vi "CaculateWaitingTimeForAlbum.vi"(9 "CurrentIndex":dbl=60000.0 format="%#_13g", 10 "ExpIncreaseEn?":bool=TRUE, 11 "Config":T1 {"Hardware Configuration"."Lasers Configuration"."SettingValues"."785 Power" format="%.1f"; "Hardware Configuration"."Lasers Configuration"."SettingValues"."647 Power" format="%.1f"; "Hardware Configuration"."Lasers Configuration"."SettingValues"."561 Power" format="%.1f"}) -> (1 "AcqTime/ms":dbl, 2 "AcqTime/min":dbl, 3 "Config 2":T1 {"Hardware Configuration"."Lasers Configuration"."SettingValues"."785 Power" format="%.1f"; "Hardware Configuration"."Lasers Configuration"."SettingValues"."647 Power" format="%.1f"; "Hardware Configuration"."Lasers Configuration"."SettingValues"."561 Power" format="%.1f"})   [LabVIEW 2019]
uses:
  Settings/System Running Settings.ctl
  Support/Hardware Configuration.ctl
  Support/Camera Configuration.ctl
  C:/RM21-MMicrosopeSource/HardwareAdapter/Camera/Dependencies/PVCamNET.dll
  Dependencies/PVCamNET.dll
  <vilib>/vision/Image Controls.llb/IMAQ Image.ctl
  C:/RM21-MMicrosopeSource/HardwareAdapter/Lasers/Dependencies/Oxxius_Boxx.dll
  Lasers/Dependencies/Oxxius_Boxx.dll
  Logging/Logging Configuration.ctl
  Controls/DeviceStatusCtl.ctl
  Controls/CallBack Refs.ctl
  Logging/Logging.lvlib
  Settings/Settings.lvlib
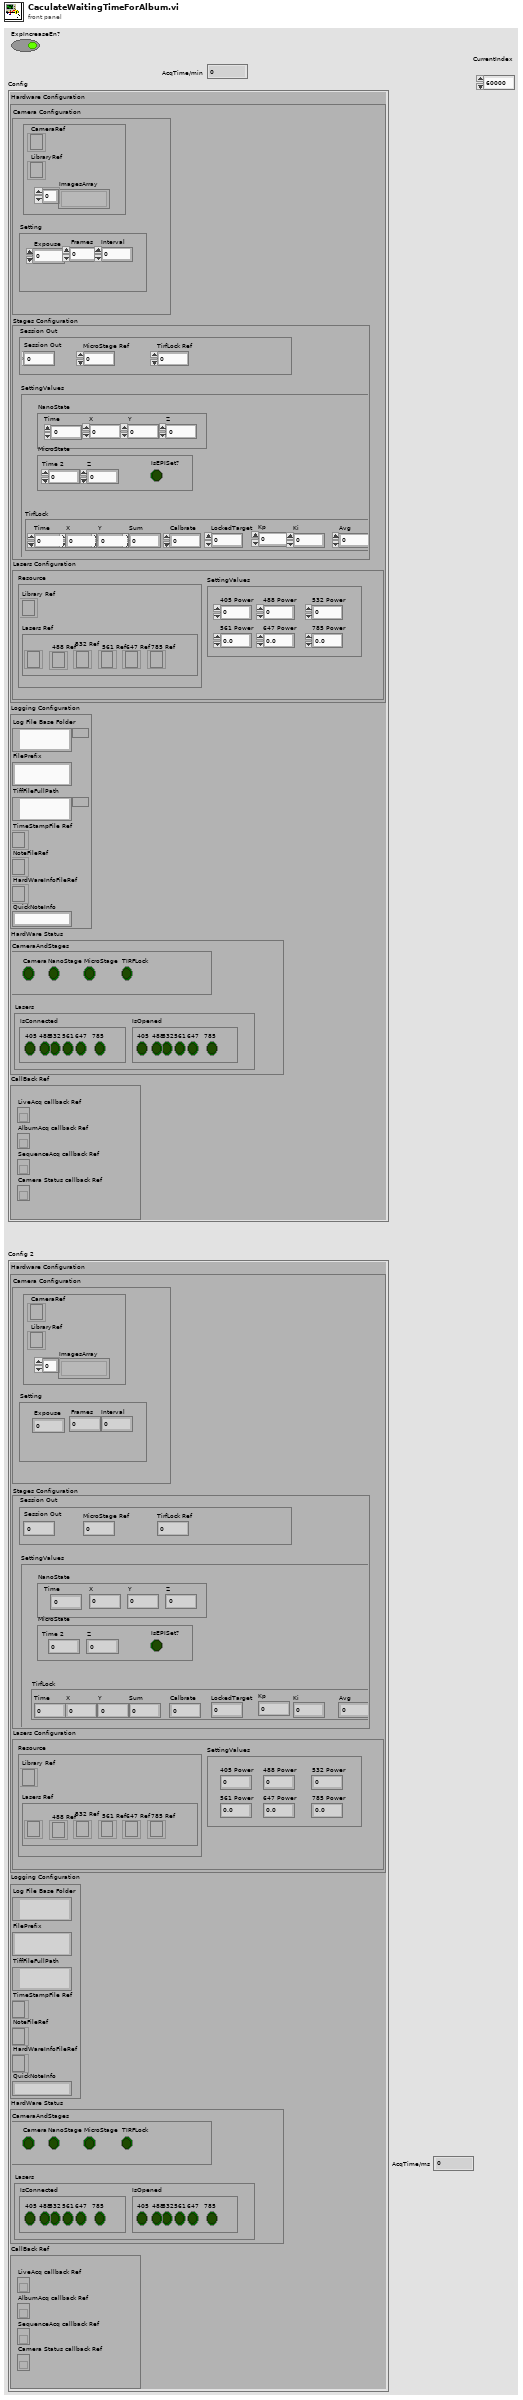
[diagram p1: front panel]
types:
  T1 = typedef "Settings.lvlib/System Running Settings.ctl" = cluster{"Hardware Configuration":T2, "Logging Configuration":T5, "HardWare Status":cluster{"CameraAndStages":T6, "Lasers":cluster{"IsConnected":cluster{"405":bool, "488":bool, "532":bool, "561":bool, "647":bool, "785":bool}, "IsOpened":cluster{"405":bool, "488":bool, "532":bool, "561":bool, "647":bool, "785":bool}}}, "CallBack Ref":T7}
  T2 = typedef "Hardware Configuration.ctl" = cluster{"Camera Configuration":T3, "Stages Configuration":cluster{"Resource":cluster{"NanoStage Ref":i32, "MicroStage Ref":i32, "TirfLock Ref":i32}, "SettingValues":cluster{"NanoState":cluster{"Time":dbl, "X":dbl, "Y":dbl, "Z":dbl}, "MicroState":cluster{"Time 2":dbl, "Z":dbl, "IsEPISet?":bool}, "TirfLock":cluster{"Time":dbl, "X":dbl, "Y":dbl, "Sum":dbl, "Calbrate":dbl, "LockedTarget":dbl, "Kp":dbl, "Ki":dbl, "Avg":dbl}}}, "Lasers Configuration":cluster{"SettingValues":cluster{"405 Power":sgl, "488 Power":sgl, "532 Power":sgl, "561 Power":sgl, "647 Power":sgl, "785 Power":sgl}, "Resource":cluster{"Library Ref":refnum<k24>, "Lasers Ref":cluster{"405 Ref":refnum<k24>, "488 Ref":refnum<k24>, "532 Ref":refnum<k24>, "561 Ref":refnum<k24>, "647 Ref":refnum<k24>, "785 Ref":refnum<k24>}}}}
  T3 = typedef "Camera Configuration.ctl" = cluster{"Setting":cluster{"Expouse":dbl, "Frames":dbl, "Interval":dbl}, "Resource":cluster{"CameraRef":refnum<k24>, "LibraryRef":refnum<k24>, "ImagesArray":T4[]}}
  T4 = typedef "IMAQ Image.ctl" = refnum<image>
  T5 = typedef "Logging.lvlib/Logging Configuration.ctl" = cluster{"Log File Base Folder":path, "FilePrefix":string, "TiffFileFullPath":path, "TimeStampFile Ref":refnum<file>, "NoteFileRef":refnum<file>, "HardWareInfoFileRef":refnum<file>, "QuickNoteInfo":string}
  T6 = typedef "DeviceStatusCtl.ctl" = cluster{"Camera":bool, "NanoStage":bool, "MicroStage":bool, "TIRFLock":bool}
  T7 = typedef "CallBack Refs.ctl" = cluster{"LiveAcq callback Ref":refnum<k27>, "AlbumAcq callback Ref":refnum<k27>, "SequenceAcq callback Ref":refnum<k27>, "Camera Status callback Ref":refnum<k27>}
  T8 = cluster{"Expouse":dbl, "Frames":dbl, "Interval":dbl}
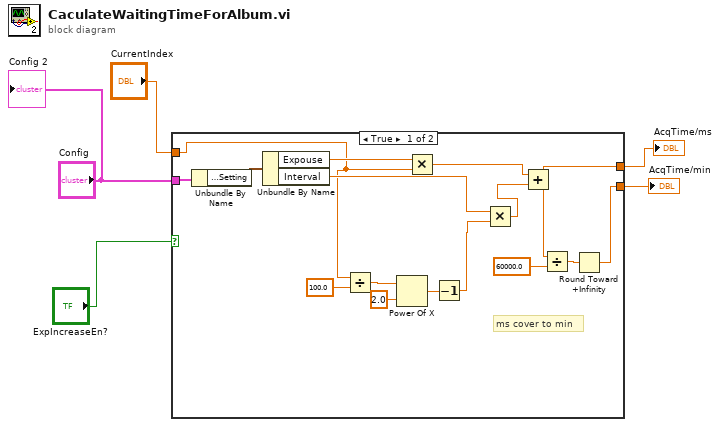
[diagram p0: block diagram]
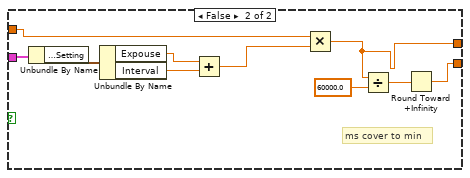
[diagram p2: hidden frame]
diagram:
  n1 = case shown="True" "ExpIncreaseEn?" {
    tunnel: "Config" -> [w21 w31]
    tunnel: [w8 w24] -> w5
    tunnel: [w7 w23] -> w2
    tunnel: "CurrentIndex" -> [w6 w22]
    frame True {
      # "ms cover to min"
      n2 = Unbundle By Name(w21) -> ("Hardware Configuration.Camera Configuration.Setting"=w20:T8)
      n3 = Unbundle By Name(w20) -> ("Expouse"=w19:dbl, "Interval"=w18:dbl)
      n4 = Divide(x=w6, y=100.0) -> (x/y=w14:dbl)
      n5 = Power Of X(1:2.0 ("x"), 2:w14) -> (0:w16:dbl)
      n6 = Multiply(x=w19, y=w6) -> (x*y=w11:dbl)
      n7 = Decrement(x=w16) -> (x-1=w15:dbl)
      n8 = Multiply(x=w18, y=w15) -> (x*y=w12:dbl)
      n9 = Add(x=w11, y=w12) -> (x+y=w7:dbl)
      n10 = Divide(x=w7, y=60000.0) -> (x/y=w9:dbl)
      n11 = Round Toward +Infinity(x=w9) -> (ceil(x): smallest int >= x=w8:dbl)
    }
    frame False {
      # "ms cover to min"
      n12 = Unbundle By Name(w31) -> ("Hardware Configuration.Camera Configuration.Setting"=w30:T8)
      n13 = Unbundle By Name(w30) -> ("Expouse"=w29:dbl, "Interval"=w28:dbl)
      n14 = Add(x=w29, y=w28) -> (x+y=w27:dbl)
      n15 = Multiply(x=w22, y=w27) -> (x*y=w23:dbl)
      n16 = Divide(x=w23, y=60000.0) -> (x/y=w25:dbl)
      n17 = Round Toward +Infinity(x=w25) -> (ceil(x): smallest int >= x=w24:dbl)
    }
  }
  "AcqTime/min" <- w5
  "AcqTime/ms" <- w2
  "Config 2" <- "Config"
